vi "De-Initialize.vi"(8 "error in (no error)":errorcluster, 11 "Delay Generator Driver in":refnum<class "Delay Generator Driver.lvclass">) -> (0 "error out":errorcluster, 3 "Delay Generator Driver out":refnum<class "Delay Generator Driver.lvclass">)   [LabVIEW 2021, in "Delay Generator Driver.lvclass"]
uses:
  Delay Generator Driver.lvclass
  Delay Generator Driver.lvclass/Delay Generator Driver.ctl
  VISA Instrument/VISA Instrument.lvclass
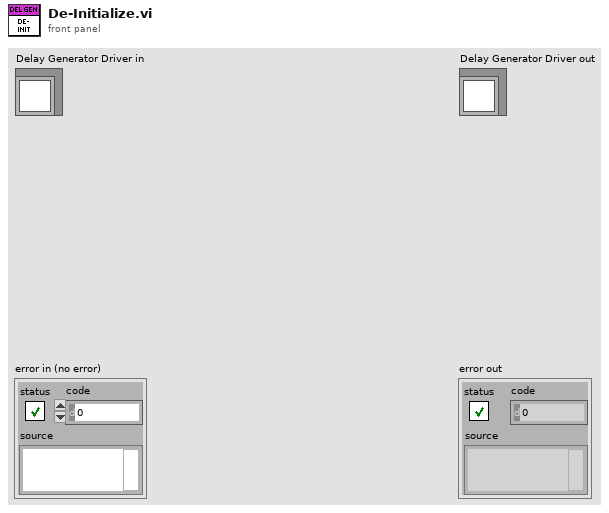
[diagram p1: front panel]
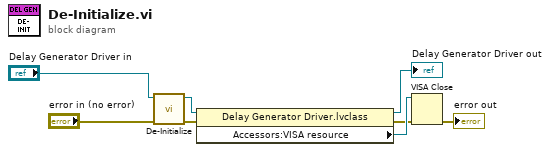
[diagram p0: block diagram]
diagram:
  n1 = call-parent "De-Initialize.vi"("error in (no error)"="error in (no error)", "Instrument Driver in"="Delay Generator Driver in") -> ("error out"=w4:errorcluster, "Instrument Driver out"=w5:refnum<class "Delay Generator Driver.lvclass">)  [unwired: 8 in]
  n2 = property class="Delay Generator Driver.lvclass"(reference=w5, error in=w4) -> (reference out=→"Delay Generator Driver out":refnum<class "Delay Generator Driver.lvclass">, error out=w2:errorcluster, "Accessors:VISA resource"=w3:refnum<visa-resource-name>)
  n3 = VISA Close(VISA resource name=w3, error in (no error)=w2) -> (error out=→"error out":errorcluster)
